vi "STArray.vi"(11 "Starting Time":u16(ring)=7 items=["AM 12:00 (mid-night)", "AM 01:00", "AM 02:00", "AM 03:00", "AM 04:00", "AM 05:00", "AM 06:00", "AM 07:00", "AM 08:00", "AM 09:00", "AM 10:00", "AM 11:00", "PM 12:00 (noon)", "PM 13:00", "PM 14:00", "PM 15:00", "PM 16:00", "PM 17:00", "PM 18:00", "PM 19:00", "PM 20:00", "PM 21:00", "PM 22:00", "PM 23:00"]) -> (0 "array w/ subset deleted":string[](array[string]), 1 "ST#(0-24)":dbl, 3 "During":u16(ring) items=["1 hour", "2 hours", "3 hours", "4 hours", "5 hours", "6 hours", "7 hours", "8 hours", "9 hours", "10 hours", "11 hours", "12 hours", "13 hours", "14 hours", "15 hours", "16 hours", "17 hours", "18 hours", "19 hours", "20 hours", "21 hours", "22 hours"])   [LabVIEW 2011]
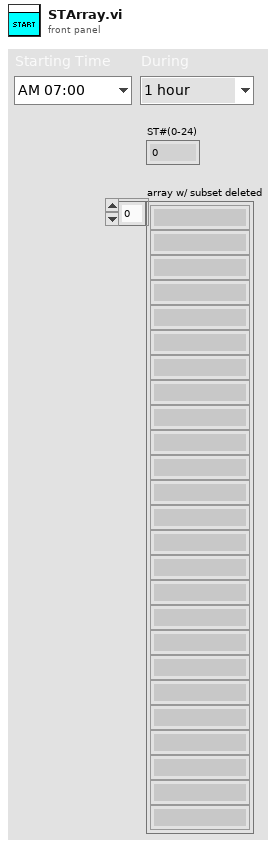
[diagram p1: front panel]
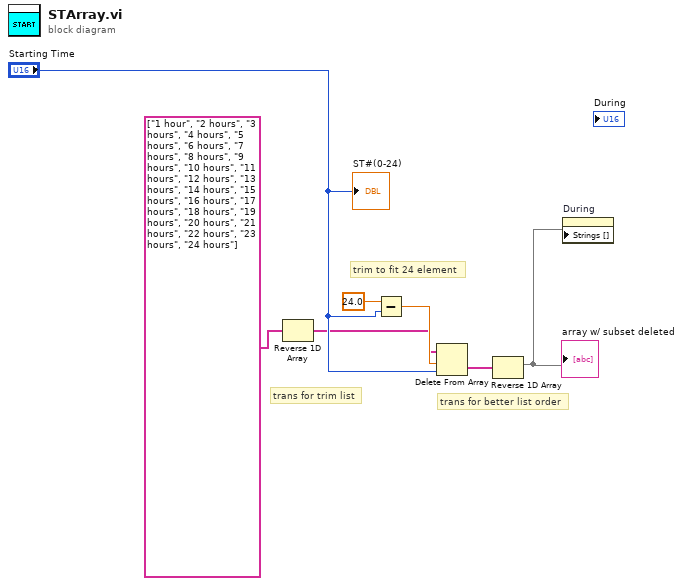
[diagram p0: block diagram]
diagram:
  # "trans for better list order"
  # "trans for trim list"
  # "trim to fit 24 element"
  n1 = Reverse 1D Array(array=string[] ["1 hour", "2 hours", "3 hours", "4 hours", "5 hours", "6 hours", "7 hours", "8 hours", "9 hours", "10 hours", "11 hours", "12 hours", "13 hours", "14 hours", "15 hours", "16 hours", "17 hours", "18 hours", "19 hours", "20 hours", "21 hours", "22 hours", "23 hours", "24 hours"]) -> (reversed array=w3:string[])
  n2 = Subtract(x=24.0, y="Starting Time") -> (x-y=w5:dbl)
  n3 = Delete From Array(array=w3, length=w5, index="Starting Time") -> (deleted portion=w2:string[])  [unwired: 1 out]
  n4 = Reverse 1D Array(array=w2) -> (reversed array=w1:string[])
  "array w/ subset deleted" <- w1
  n5 = property on="During" class="Ring (strict)"("Strings []"=w1) -> ()  [unwired: 2 in, 2 out]
  "ST#(0-24)" <- "Starting Time"
